vi "enqueueElem.vi"(8 "error_in":errorcluster, 10 "element":T1, 11 "queue_in":refnum<queue>) -> (0 "error_out":errorcluster, 3 "queue_out":refnum<queue>)   [LabVIEW 2017]
uses:
  controls/stateMachine.ctl
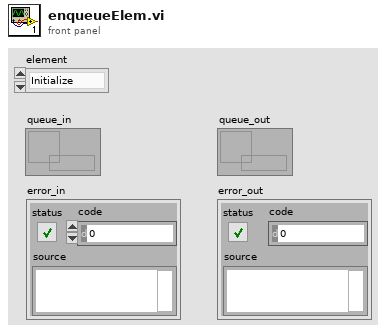
[diagram p1: front panel]
types:
  T1 = typedef "stateMachine.ctl" = enum16{"Initialize", "Start", "Pause", "Stop", "Shutdown"}
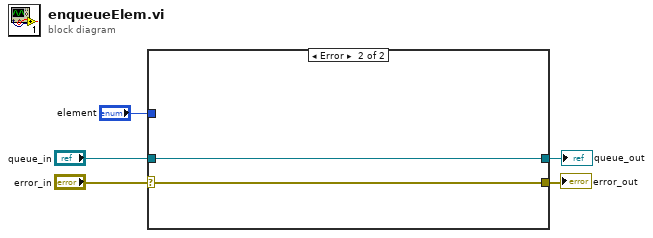
[diagram p0: block diagram]
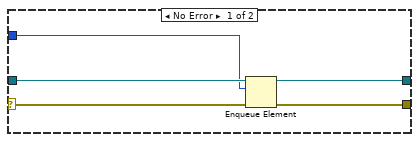
[diagram p2: hidden frame]
diagram:
  n1 = case shown="Error" "error_in" {
    selector: "error_in" -> [w10 w12]
    tunnel: [w9 w12] -> w1
    tunnel: [w8 w11] -> w2
    tunnel: "queue_in" -> [w7 w11]
    tunnel: "element" -> [w6 _]
    frame No Error {
      n2 = Enqueue Element(queue=w7, element=w6, error in (no error)=w10) -> (queue out=w8:refnum<queue>, error out=w9:errorcluster)  [unwired: 1 in, 1 out]
    }
    frame Error {
    }
  }
  "queue_out" <- w2
  "error_out" <- w1
